vi "log sent message.vi"(8 "error in (no error)":errorcluster, 11 "Socket in":refnum<class "Socket.lvclass">) -> (0 "error out":errorcluster, 3 "Socket out":refnum<class "Socket.lvclass">)   [LabVIEW 2018, in "Socket.lvclass"]
uses:
  Socket.lvclass
  Socket.lvclass/Socket.ctl
  Log File/CM_Log File.lvclass
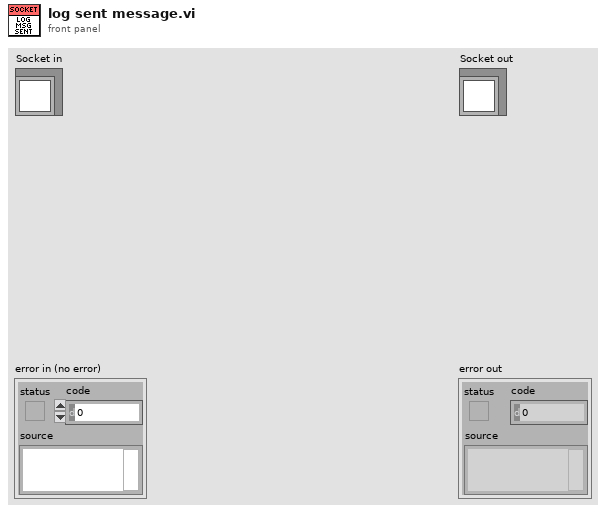
[diagram p1: front panel]
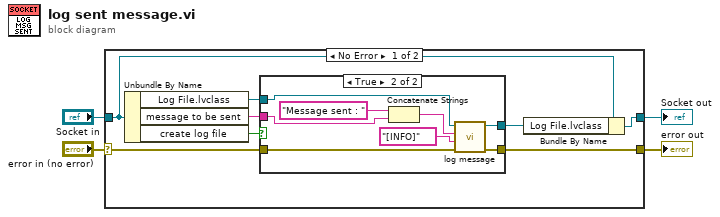
[diagram p0: block diagram]
diagram:
  n1 = case shown="No Error" "error in (no error)" {
    selector: "error in (no error)" -> [w10 w24]
    tunnel: [w9 w24] -> w3
    tunnel: [w5 w23] -> w1
    tunnel: "Socket in" -> [w7 w23]
    frame No Error {
      n2 = Unbundle By Name(w7) -> ("Log File.lvclass"=w8:refnum<class "CM_Log File.lvclass">, "message to be sent"=w11:string, "create log file"=w12:bool)
      n3 = case shown="True" w12 {
        tunnel: w11 -> [_ w17]
        tunnel: w10 -> [w14 w21]
        tunnel: [w14 w20] -> w9
        tunnel: w8 -> [w13 w19]
        tunnel: [w13 w18] -> w6
        frame False {
        }
        frame True {
          n4 = Concatenate Strings("Message sent : " ("string"), w17) -> (w16:string)
          n5 = call-dynamic "log message.vi"("error in (no error)"=w21, "message type"="[INFO]", "Message to log"=w16, "Log File in"=w19) -> ("error out"=w20:errorcluster, "Log File out"=w18:refnum<class "CM_Log File.lvclass">)  [unwired: 6 in]
        }
      }
      n6 = Bundle By Name(cluster=w7, "Log File.lvclass"=w6) -> (w5:refnum<class "Socket.lvclass">)
    }
    frame Error {
    }
  }
  "error out" <- w3
  "Socket out" <- w1
